vi "SngJntArmSim_Update.vi"(10 "dT_Seconds":dbl=1.0, 11 "in SingleJointArmSim":T1 {"GearBox"."Jr_KgM2" format="%13.5p"; "GearBox"."L_H" format="%13.5p"; "GearBox"."Kt_NMPerAmp" format="%13.5p"; "GearBox"."KvINV_RadPerSecPerVolt" format="%13.5p"; "GearBox"."R_Ohms" format="%13.5p"; "GearBox"."FreeSpeed_RadPerSec" format="%13.5p"; "GearBox"."FreeCurrent_Amps" format="%13.5p"; "GearBox"."StallCurrent_Amps" format="%13.5p"; "GearBox"."StallTorque_NM" format="%13.5p"; "GearBox"."nominalVoltage_Volts" format="%13.5p"}) -> (0 "Error":bool, 3 "out SingleJointArmSim":T1 {"GearBox"."Jr_KgM2" format="%13.5p"; "GearBox"."L_H" format="%13.5p"; "GearBox"."Kt_NMPerAmp" format="%13.5p"; "GearBox"."KvINV_RadPerSecPerVolt" format="%13.5p"; "GearBox"."R_Ohms" format="%13.5p"; "GearBox"."FreeSpeed_RadPerSec" format="%13.5p"; "GearBox"."FreeCurrent_Amps" format="%13.5p"; "GearBox"."StallCurrent_Amps" format="%13.5p"; "GearBox"."StallTorque_NM" format="%13.5p"; "GearBox"."nominalVoltage_Volts" format="%13.5p"})   [LabVIEW 2019, in "Trajectory_Library.lvlib"]
doc: "Updates the simulation.\n \nInputs:\n - SngJntArmSim -- Data cluster\n - dtSeconds -- The time between updates.\n\nOutputs:\n - OutSngJntArmSim -- Updated data cluster\n - Error -- If TRUE, an error occured."
uses:
  Trajectory_Library.lvlib
  SINGLE_JOINT_ARM_SIM.ctl
  LINEAR_SYSTEM_SIM.ctl
  LINEAR_SYSTEM.ctl
  <vilib>/Analysis/Matrix/Datatypes/RealMatrix.ctl
  DCMOTOR.CTL
  <vilib>/Analysis/Matrix/NI_Matrix.lvlib
panel:
  # "<1, 1>"
  # "<States, 1>"
  # "<Outputs, 1>"
  # "<Inputs, 1>"
  # "<Outputs, 1>"
  # "<States,States>"
  # "<States,Inputs>"
  # "<Outputs,States>"
  # "<Outputs,Inputs>"
  # "<States, 1>"
  # "<Outputs, 1>"
  # "<Inputs, 1>"
  # "<Outputs, 1>"
  # "<States,States>"
  # "<States,Inputs>"
  # "<Outputs,States>"
  # "<Outputs,Inputs>"
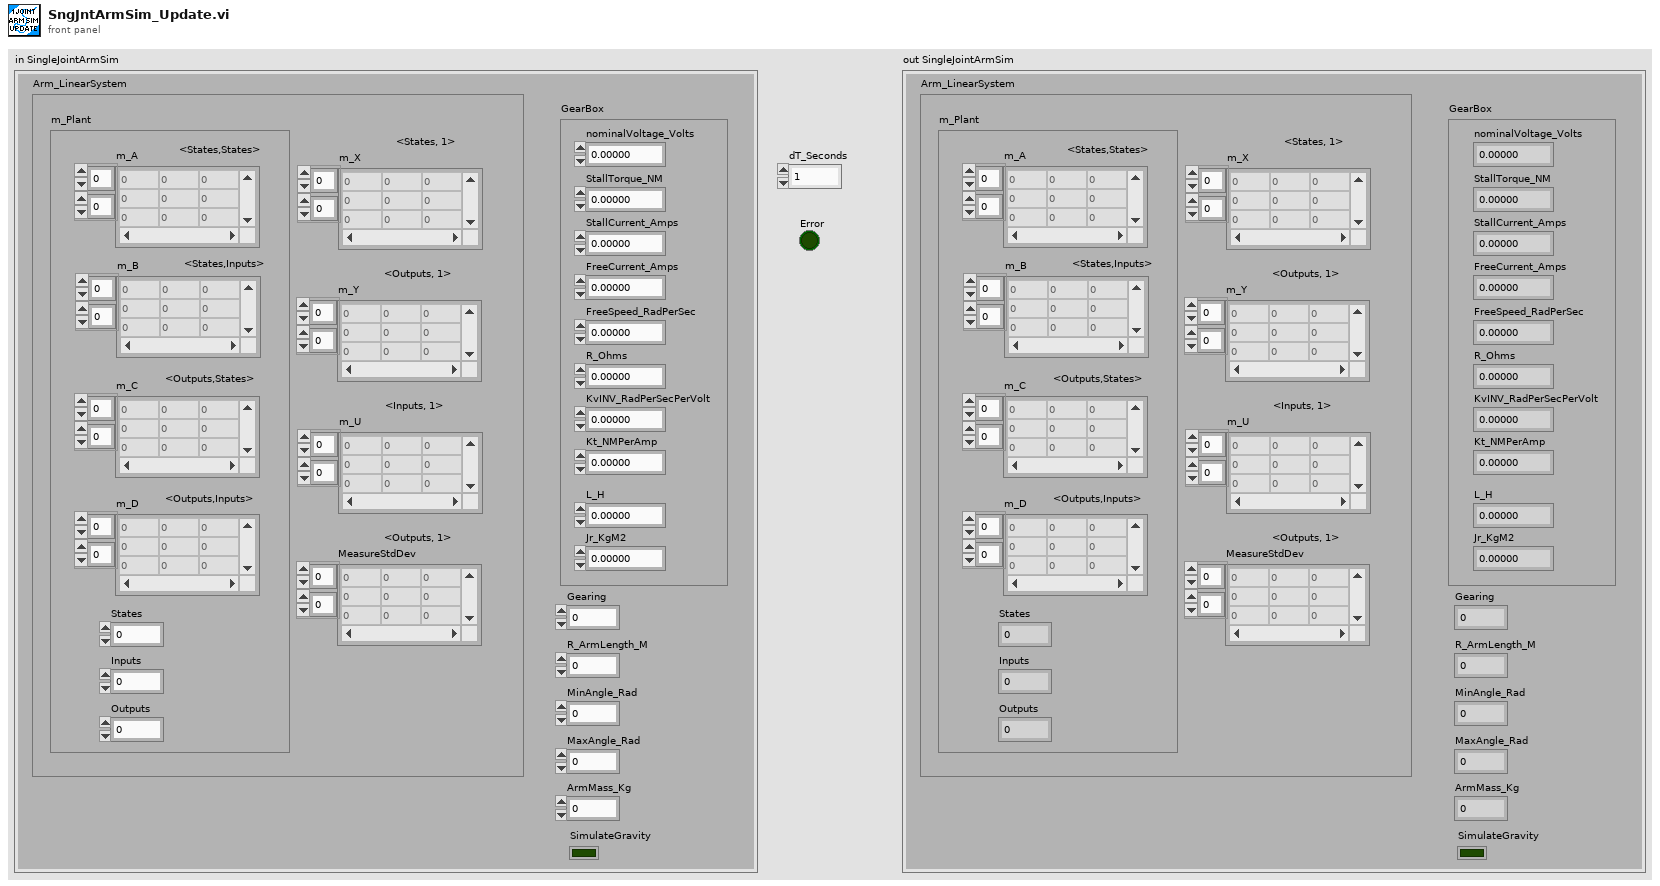
[diagram p1: front panel]
types:
  T1 = typedef "Trajectory_Library.lvlib/SINGLE_JOINT_ARM_SIM.ctl" = cluster{"Arm_LinearSystem":T2, "GearBox":T5, "Gearing":dbl, "R_ArmLength_M":dbl, "MinAngle_Rad":dbl, "MaxAngle_Rad":dbl, "ArmMass_Kg":dbl, "SimulateGravity":bool}
  T2 = typedef "Trajectory_Library.lvlib/LINEAR_SYSTEM_SIM.ctl" = cluster{"m_Plant":T3, "m_X":T4, "m_Y":T4, "m_U":T4, "MeasureStdDev":T4}
  T3 = typedef "Trajectory_Library.lvlib/LINEAR_SYSTEM.ctl" = cluster{"m_A":T4, "m_B":T4, "m_C":T4, "m_D":T4, "States":i32, "Inputs":i32, "Outputs":i32}
  T4 = typedef "NI_Matrix.lvlib/RealMatrix.ctl" = dbl[][]
  T5 = typedef "Trajectory_Library.lvlib/DCMOTOR.CTL" = cluster{"nominalVoltage_Volts":dbl, "StallTorque_NM":dbl, "StallCurrent_Amps":dbl, "FreeCurrent_Amps":dbl, "FreeSpeed_RadPerSec":dbl, "R_Ohms":dbl, "KvINV_RadPerSecPerVolt":dbl, "Kt_NMPerAmp":dbl, "L_H":dbl, "Jr_KgM2":dbl}
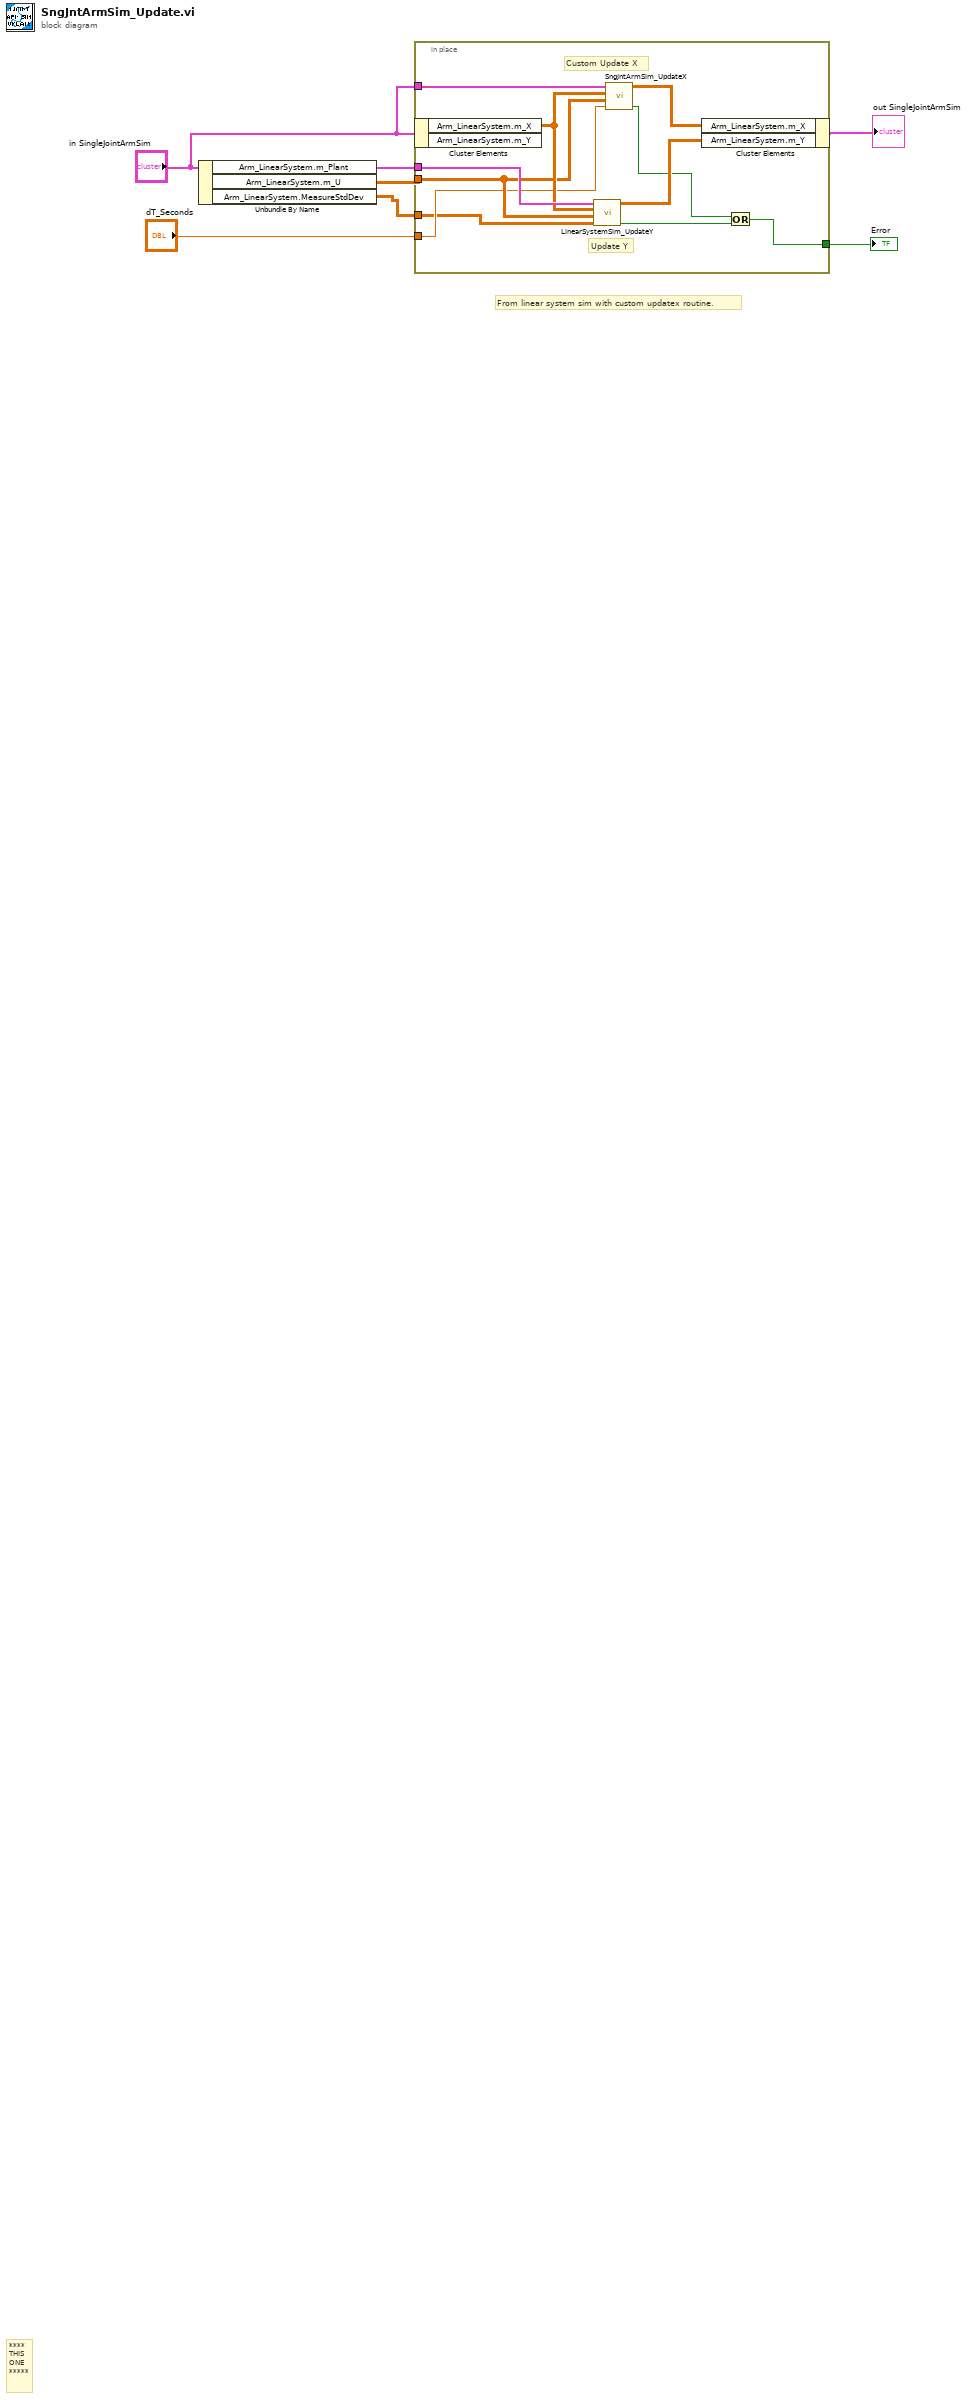
[diagram p0: block diagram]
diagram:
  # "From linear system sim with custom updatex routine."
  # "****\nTHIS\nONE\n*****"
  n1 = Unbundle By Name("in SingleJointArmSim") -> ("Arm_LinearSystem.m_Plant"=w4:T3, "Arm_LinearSystem.m_U"=w5:T4, "Arm_LinearSystem.MeasureStdDev"=w2:T4)
  n2 = in-place {
    in-place-border: w5 -> [w14]
    in-place-border: "dT_Seconds" -> [w13]
    in-place-border: "in SingleJointArmSim" -> [w12]
    in-place-border: w4 -> [w17]
    in-place-border: w2 -> [w11]
    in-place-border: [w8] -> w1
    # "Update Y"
    # "Custom Update X"
    n3 = in-place-cluster #1("in SingleJointArmSim") -> ("Arm_LinearSystem.m_X"=w15:T4)  [unwired: 1 out]
    n4 = call "LinearSystemSim_UpdateY.vi"("MeasurementStdDev"=w11, "ClampedU"=w14, "X"=w15, "Linearsystem"=w17) -> ("Error"=w9:bool, "Y"=w18:T4)  [unwired: 6 in]
    n5 = call "SngJntArmSim_UpdateX.vi"("dT_Seconds"=w13, "U"=w14, "current_xHat"=w15, "SINGLE_JOINT_ARM_SIM"=w12) -> ("Error"=w10:bool, "updated_xHat"=w16:T4)  [unwired: 6 in]
    n6 = in-place-cluster #1("Arm_LinearSystem.m_X"=w16, "Arm_LinearSystem.m_Y"=w18) -> (→"out SingleJointArmSim":T1)
    n7 = Or(x=w10, y=w9) -> (x .or. y?=w8:bool)
  }
  "Error" <- w1
